vi "ShowData.vi"(7 "subchannel":i32, 11 "data in":refnum<class "EventMessengerMData.lvclass">) -> (0 "aborted?":bool, 2 "write count":u32, 3 "data out":refnum<class "EventMessengerMData.lvclass">, 4 "last element?":bool)   [LabVIEW 2019, in "Event MessengerM.lvlib" / "EventMessengerMData.lvclass"]
uses:
  EventMessengerMData.lvclass
  EventMessengerMData.lvclass/EventMessengerMData.ctl
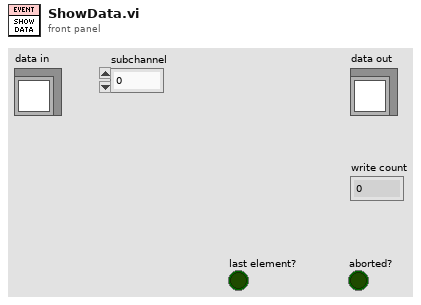
[diagram p1: front panel]
types:
  T1 = map{i32, cluster{"Write Count":u32, "Reg Refnum":u32, "aborted?":bool, "last element?":bool, "Event Refnum":refnum<user-event>}}
  T2 = cluster{"Write Count":u32, "Reg Refnum":u32, "aborted?":bool, "last element?":bool, "Event Refnum":refnum<user-event>}
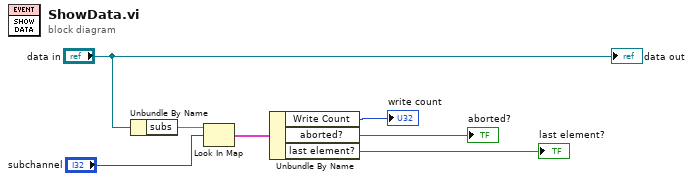
[diagram p0: block diagram]
diagram:
  n1 = Unbundle By Name("data in") -> ("subs"=w2:T1)
  n2 = Look In Map(map=w2, key="subchannel") -> (value=w3:T2)  [unwired: 1 in, 1 out]
  n3 = Unbundle By Name(w3) -> ("Write Count"=→"write count":u32, "aborted?"=→"aborted?":bool, "last element?"=→"last element?":bool)
  "data out" <- "data in"
